vi "Draw Current Position Marker.vi"(8 "Error In (no Error) In":errorcluster, 10 "Current Location In":i32, 11 "Array In":T1[](array[typedef])) -> (0 "Error Out":errorcluster, 3 "Array Out":T1[](array[typedef]))   [LabVIEW 2018, in "Waveform Control.xctl"]
doc: "Generates a waveform that is NaN apart from the one point at the given index position. The Y value of this point is the same as the corresponding point in the first waveform of the array input,"
uses:
  Waveform Control.xctl
  Controls/Data.ctl
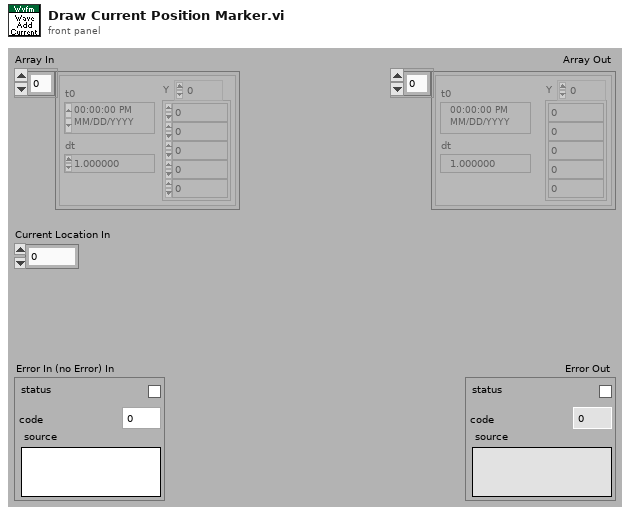
[diagram p1: front panel]
types:
  T1 = typedef "Waveform Control.xctl/Data.ctl" = waveform(dbl)
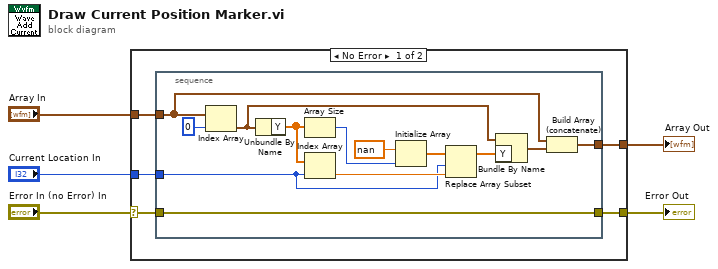
[diagram p0: block diagram]
diagram:
  n1 = case shown="No Error" "Error In (no Error) In" {
    selector: "Error In (no Error) In" -> [w6 w24]
    tunnel: [w10 _] -> w5
    tunnel: "Array In" -> [w9 _]
    tunnel: "Current Location In" -> [w8 _]
    tunnel: [w7 w24] -> w2
    frame No Error {
      n2 = stacked-sequence {
        tunnel: [w23] -> w10
        tunnel: w9 -> [w21]
        tunnel: w8 -> [w12]
        tunnel: [w11] -> w7
        tunnel: w6 -> [w11]
        frame #0 {
          n3 = Index Array(array=w21, index=0) -> (element=w20:T1)
          n4 = Unbundle By Name(w20) -> ("Y"=w17:dbl[])
          n5 = Array Size(array=w17) -> (size(s)=w14:i32)
          n6 = Index Array(array=w17, index=w12) -> (element=w18:dbl)
          n7 = Initialize Array(nan ("element"), w14) -> (w16:dbl[])
          n8 = Replace Array Subset(array=w16, new element=w18, index=w12) -> (w19:dbl[])
          n9 = Bundle By Name(cluster=w20, "Y"=w19) -> (w22:T1)
          n10 = Build Array (concatenate)(w21, w22) -> (w23:T1[])
        }
      }
    }
    frame Error {
    }
  }
  "Array Out" <- w5
  "Error Out" <- w2
